vi "Set VI Icon.vi"(10 "路径":path, 11 "VI引用句柄":refnum<vi>) -> (2 "OldHandle":u32, 3 "ImageHandle":u32)   [LabVIEW 2013]
uses:
  USER32.DLL
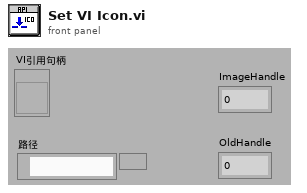
[diagram p1: front panel]
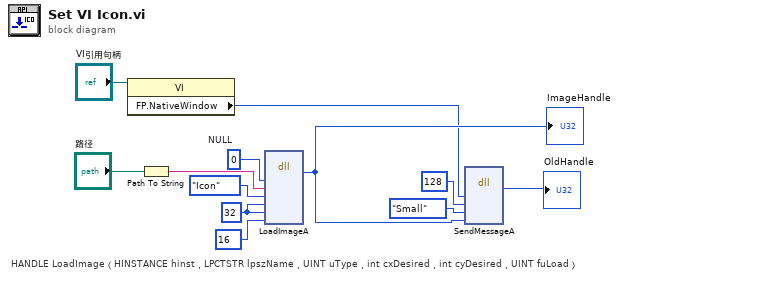
[diagram p0: block diagram]
diagram:
  w11 = u32 32 ("cxDesired")
  w12 = u32 0  # NULL
  # "HANDLE LoadImage（HINSTANCE hinst，LPCTSTR lpszName，UINT uType，int cxDesired，int cyDesired，UINT fuLoad）"
  n1 = property class="VI"(reference="VI引用句柄") -> ("FP.NativeWindow"=w2:u64)  [unwired: 1 in, 2 out]
  n2 = Path To String(path="路径") -> (string=w9:string)
  n3 = dll-call lib="user32.dll" fn="LoadImageA" label="LoadImage"("HINSTANCE"=w12, "LPCTSTR"=w9, "uType"=enum16{"Bitmap", "Icon", "Cursor"}."Icon", "cxDesired"=w11, "cyDesired"=w11, "fuLoad"=16) -> ("ImageHandle"=w4:u32)  [unwired: 9 in, 2 out]
  "ImageHandle" <- w4
  n4 = dll-call lib="user32.dll" fn="SendMessageA" label="SendMessage"("hWnd"=w2, "uMsg"=u32 128 ("dimension size"), "wParam"=enum16{"Small", "Big"}."Small", "lParam"=w4) -> ("OldHandle"=→"OldHandle":u32)  [unwired: 7 in, 2 out]
